vi "parse US data.vi"(9 "Error message":string="Error downloading file", 10 "has population values":bool, 11 "URL":string="https://raw.githubusercontent.com/CSSEGISandData/COVID-19/master/csse_covid_19_data/csse_covid_19_time_series/time_series_covid19_deaths_US.csv") -> (0 "populations":i32[](array[numeric]), 1 "Array 3":string[](array[string]), 2 "per day":i32[][](array[numeric]), 3 "cumulative":i32[][](array[numeric]))   [LabVIEW 2019]
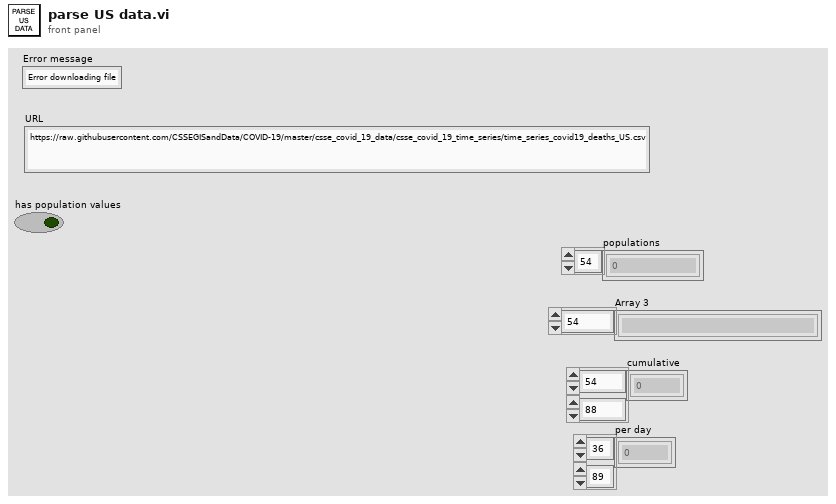
[diagram p1: front panel]
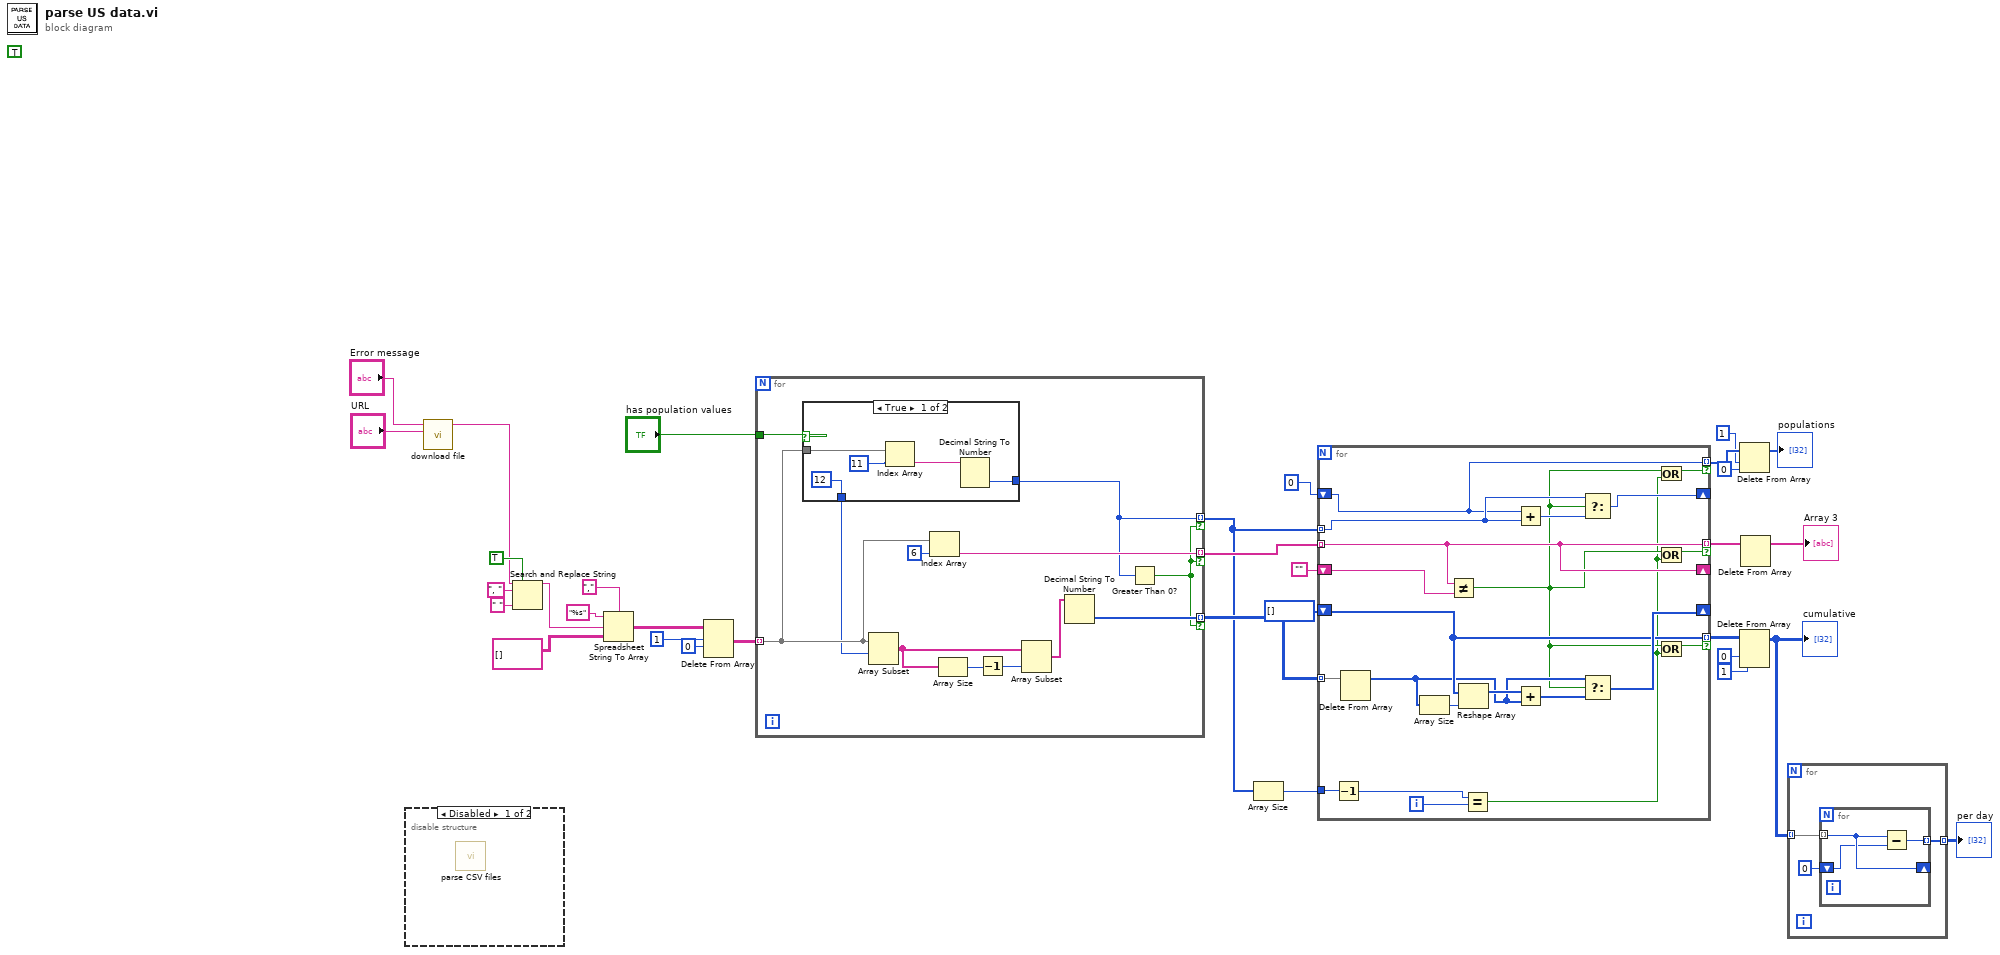
[diagram p0: block diagram]
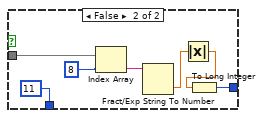
[diagram p3: hidden frame]
diagram:
  (unwired) TRUE
  n1 = disable-structure shown="Disabled" {
    frame Disabled {
      n2 = call "parse CSV files.vi"() -> ()  [unwired: 6 in, 6 out]
    }
    frame Enabled {
    }
  }
  n3 = call "download file.vi"("URL"="URL", "Error message"="Error message") -> ("downloaded file"=w3:string)  [unwired: 8 in, 1 out]
  n4 = Search and Replace String(replace all?=TRUE ("replace all? (F)"), input string=w3, search string=", ", replace string=" " ("replace string (\"\")")) -> (result string=w23:string)  [unwired: 4 in, 3 out]
  n5 = Spreadsheet String To Array(delimiter (Tab)=",", format string="%s", spreadsheet string=w23, array type (2D Dbl)=string[][] []) -> (array=w29:string[][])
  n6 = Delete From Array(array=w29, length=1, index (row)=0) -> (array with subset deleted=w30:string[][])  [unwired: 1 in, 1 out]
  n7 = for {
    tunnel: w30 -> [w38] mode=indexing
    tunnel: [w40] -> w21 mode=indexing if=w36
    tunnel: [w39] -> w22 mode=indexing if=w36
    tunnel: [w37] -> w10 mode=indexing if=w36
    tunnel: "has population values" -> [w35]
    n8 = case shown="True" w35 {
      tunnel: w38 -> [w49 w56]
      tunnel: [w47 w54] -> w37
      tunnel: [12 ("index") 11 ("index")] -> w34
      frame True {
        n9 = Index Array(array=w49, index=11) -> (element=w48:string)
        n10 = Decimal String To Number(string=w48) -> (number=w47:i32)  [unwired: 2 in, 1 out]
      }
      frame False {
        n11 = Index Array(array=w56, index=8) -> (element=w55:string)
        n12 = Fract/Exp String To Number(string=w55) -> (number=w52:dbl)  [unwired: 3 in, 1 out]
        n13 = Absolute Value(x=w52) -> (abs(x)=w51:dbl)
        n14 = To Long Integer(number=w51) -> (32bit integer=w54:i32)
      }
    }
    n15 = Array Subset(array=w38, index=w34) -> (w44:string[])  [unwired: 1 in]
    n16 = Index Array(array=w38, index=6) -> (element=w39:string)
    n17 = Array Size(array=w44) -> (size(s)=w43:i32)
    n18 = Decrement(x=w43) -> (x-1=w45:i32)
    n19 = Array Subset(array=w44, length=w45) -> (w42:string[])  [unwired: 1 in]
    n20 = Decimal String To Number(string=w42) -> (number=w40:i32[])  [unwired: 2 in, 1 out]
    n21 = Greater Than 0?(x=w37) -> (x > 0?=w36:bool)
  }
  n22 = Array Size(array=w10) -> (size(s)=w9:i32)
  n23 = for {
    tunnel: w22 -> [w77] mode=indexing
    tunnel: w21 -> [w71] mode=indexing
    shift-right: [w77] -> _
    shift-left: "" -> [w78]
    shift-right: [w76] -> _
    shift-left: i32[] [] -> [w72]
    tunnel: [w72] -> w18 mode=indexing if=w62
    tunnel: [w77] -> w7 mode=indexing if=w63
    tunnel: w10 -> [w68] mode=indexing
    shift-right: [w67] -> _
    shift-left: 0 -> [w66]
    tunnel: [w66] -> w14 mode=indexing if=w64
    tunnel: w9 -> [w60]
    i -> [w61]
    n24 = Decrement(x=w60) -> (x-1=w59:i32)
    n25 = Delete From Array(array=w71) -> (array with subset deleted=w70:i32[])  [unwired: 2 in, 1 out]
    n26 = Array Size(array=w70) -> (size(s)=w73:i32)
    n27 = Not Equal?(x=w77, y=w78) -> (x != y?=w65:bool)
    n28 = Reshape Array(w72, w73) -> (w74:i32[])
    n29 = Equal?(x=w59, y=w61) -> (x = y?=w58:bool)
    n30 = Add(x=w66, y=w68) -> (x+y=w69:i32)
    n31 = Add(x=w74, y=w70) -> (x+y=w75:i32[])
    n32 = Select(t=w68, s=w65, f=w69) -> (s? t:f=w67:i32)
    n33 = Select(t=w70, s=w65, f=w75) -> (s? t:f=w76:i32[])
    n34 = Or(x=w65, y=w58) -> (x .or. y?=w64:bool)
    n35 = Or(x=w65, y=w58) -> (x .or. y?=w63:bool)
    n36 = Or(x=w65, y=w58) -> (x .or. y?=w62:bool)
  }
  n37 = Delete From Array(array=w14, length=1, index=0 ("index (row)")) -> (array with subset deleted=→"populations":i32[])  [unwired: 1 out]
  n38 = Delete From Array(array=w18, length=1, index (row)=0) -> (array with subset deleted=w6:i32[][])  [unwired: 1 in, 1 out]
  "cumulative" <- w6
  n39 = Delete From Array(array=w7) -> (array with subset deleted=→"Array 3":string[])  [unwired: 2 in, 1 out]
  n40 = for {
    tunnel: [w80] -> w5 mode=indexing
    tunnel: w6 -> [w79] mode=indexing
    n41 = for {
      tunnel: w79 -> [w84] mode=indexing
      shift-right: [w84] -> _
      shift-left: 0 -> [w83]
      tunnel: [w82] -> w80 mode=indexing
      n42 = Subtract(x=w84, y=w83) -> (x-y=w82:i32)
    }
  }
  "per day" <- w5
